vi "Configure Device.vi"(8 "error in (no error)":errorcluster, 11 "CPC in":refnum<class "CPC.lvclass">) -> (0 "error out":errorcluster, 3 "CPC out":refnum<class "CPC.lvclass">)   [LabVIEW 2014, in "CPC.lvclass"]
uses:
  CPC.lvclass
  reusable/Session APIs/Serial/Serial Session.lvclass
  <vilib>/Utility/config.llb/NI_LVConfig.lvlib
  <vilib>/Utility/config.llb/Read Key (Boolean).vi
  reusable/Session APIs/File Access/Config Data/Config Data.lvclass
  reusable/Session APIs/Serial/Typedefs/Serial Config.ctl
  reusable/Session APIs/Serial/Typedefs/Msg Config.ctl
  <vilib>/Utility/config.llb/Read Key (String).vi
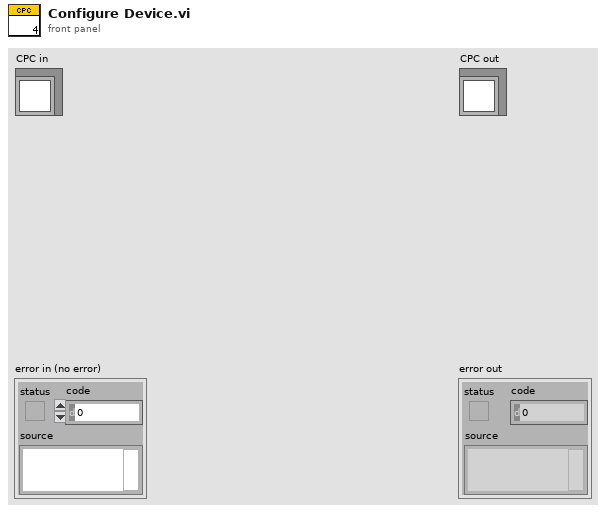
[diagram p1: front panel]
types:
  T1 = typedef "Serial Session.lvclass/Msg Config.ctl" = cluster{"sendEndEn":bool, "suppEnEnRd":bool, "termChar":u8, "EnTermChar":bool}
  T2 = typedef "Serial Session.lvclass/Serial Config.ctl" = cluster{"baud rate":u32, "data bits":u16, "stop bits":u16, "parity":u16, "flow control":u16, "endModeforReads":u16, "endModeforWrites":u16}
  T3 = typedef "Config Data.lvclass/Config Session.ctl" = refnum<data-value>
  T4 = typedef "NI_LVConfig.lvlib/Config Data RefNum.ctl" = refnum<k1>
  T5 = typedef "Serial Session.lvclass/Session Handle.ctl" = refnum<data-value>
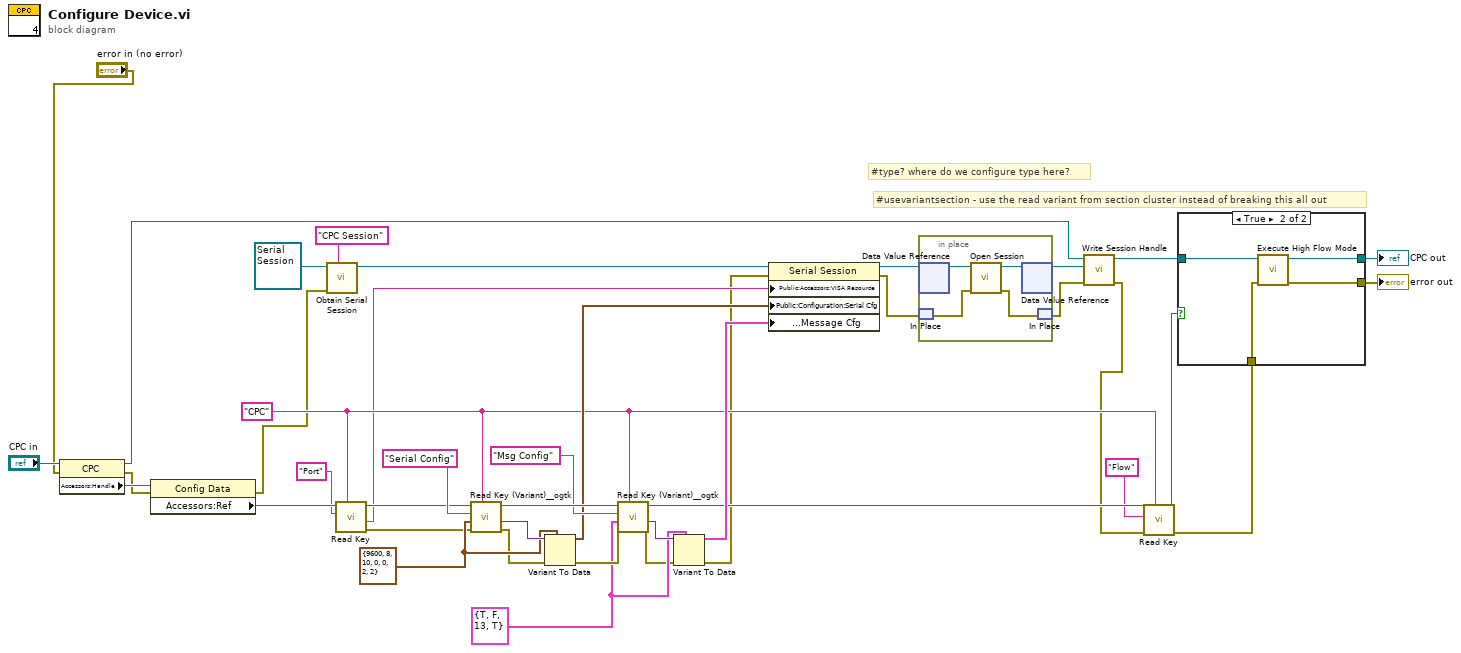
[diagram p0: block diagram]
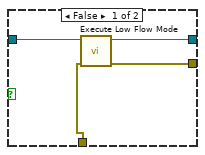
[diagram p2: hidden frame]
diagram:
  w28 = T1 {"sendEndEn"=TRUE, "suppEnEnRd"=FALSE, "termChar"=13, "EnTermChar"=TRUE} ("Msg Configuration")
  w33 = T2 {"baud rate"=9600, "data bits"=8, "stop bits"=10, "parity"=0, "flow control"=0, "endModeforReads"=2, "endModeforWrites"=2} ("Serial Config")
  w18 = "CPC" ("section")
  # "#usevariantsection - use the read variant from section cluster instead of breaking this all out"
  # "#type? where do we configure type here?"
  n1 = property class="CPC"(reference="CPC in", error in="error in (no error)") -> (reference out=w12:refnum<class "CPC.lvclass">, error out=w8:errorcluster, "Accessors:Handle"=w36:T3)
  n2 = property class="Config Data"(reference=w36, error in=w8) -> (error out=w7:errorcluster, "Accessors:Ref"=w23:T4)  [unwired: 1 out]
  n3 = call "Obtain Serial Session.vi"("Session Name ()"="CPC Session", "error in"=w7, "Serial Session in"=refnum<class "Serial Session.lvclass"> refnum) -> ("hSerial"=w38:T5)  [unwired: 6 in, 2 out]
  n4 = call-poly <vilib>:"Read Key.vi"("section"=w18, "key"="Port" ("section"), "refnum"=w23) -> ("error out"=w24:errorcluster, "value"=w16:string, "refnum out"=w25:T4)  [unwired: 5 in, 1 out]
  n5 = call <userlib>:"Read Key (Variant)__ogtk.vi"("section"=w18, "error in (no error)"=w24, "type"=w33, "key (optional)"="Serial Config", "refnum"=w25) -> ("error out"=w22:errorcluster, "key-value"=w34:variant, "refnum out"=w32:T4)  [unwired: 3 in, 1 out]
  n6 = Variant To Data(error in=w22, type=w33, Variant=w34) -> (data=w27:T2, error out=w31:errorcluster)
  n7 = call <userlib>:"Read Key (Variant)__ogtk.vi"("section"=w18, "error in (no error)"=w31, "type"=w28, "key (optional)"="Msg Config", "refnum"=w32) -> ("error out"=w21:errorcluster, "key-value"=w29:variant, "refnum out"=w20:T4)  [unwired: 3 in, 1 out]
  n8 = Variant To Data(error in=w21, type=w28, Variant=w29) -> (data=w26:T1, error out=w9:errorcluster)
  n9 = property class="Serial Session"(reference=w38, error in=w9, "Public:Accessors:VISA Resource"=w16, "Public:Configuration:Serial Cfg"=w27, "Public:Configuration:Message Cfg"=w26) -> (reference out=w15:T5, error out=w14:errorcluster)
  n10 = in-place {
    n11 = in-place-dvr #1(w15) -> (w44:refnum<class "Serial Session.lvclass">)  [unwired: 1 out]
    n12 = in-place-match #2(w14) -> (w43:errorcluster)
    n13 = call "Open Session.vi"("error in (no error)"=w43, "Serial Session in"=w44) -> ("error out"=w42:errorcluster, "Serial Session out"=w41:refnum<class "Serial Session.lvclass">)  [unwired: 8 in]
    n14 = in-place-dvr #1(w41) -> (w13:T5)  [unwired: 1 out]
    n15 = in-place-match #2(w42) -> (w6:errorcluster)
  }
  n16 = call "Write Session Handle.vi"("error in"=w6, "Session Handle"=w13, "CPC in"=w12) -> ("error out"=w5:errorcluster, "CPC out"=w11:refnum<class "CPC.lvclass">)  [unwired: 7 in]
  n17 = call-poly <vilib>:"Read Key.vi"("section"=w18, "error in (no error)"=w5, "key"="Flow", "refnum"=w20) -> ("error out"=w4:errorcluster, "value"=w10:bool)  [unwired: 4 in, 2 out]
  n18 = case shown="True" w10 {
    tunnel: w11 -> [w48 w52]
    tunnel: w4 -> [w45 w51]
    tunnel: [w46 w50] -> w1
    tunnel: [w47 w49] -> w3
    frame False {
      n19 = call "Execute Low Flow Mode.vi"("error in"=w45, "CPC in"=w48) -> ("error out"=w46:errorcluster, "CPC out"=w47:refnum<class "CPC.lvclass">)  [unwired: 7 in, 1 out]
    }
    frame True {
      n20 = call "Execute High Flow Mode.vi"("error in"=w51, "CPC in"=w52) -> ("error out"=w50:errorcluster, "CPC out"=w49:refnum<class "CPC.lvclass">)  [unwired: 7 in, 1 out]
    }
  }
  "error out" <- w1
  "CPC out" <- w3
